vi "Group Modules.vi"(8 "error in":errorcluster, 10 "Item Names":string[](array[string]), 11 "json class out":refnum<class "Build_Javier_Lopez_lib_Configuration_Filejson class.lvclass">) -> (0 "error out":errorcluster, 2 "Enum":T1(c390))   [LabVIEW 2021]
uses:
  <vilib>/Javier Lopez/Configuration File/Json Element/Build_Javier_Lopez_lib_Configuration_Filejson class.lvclass
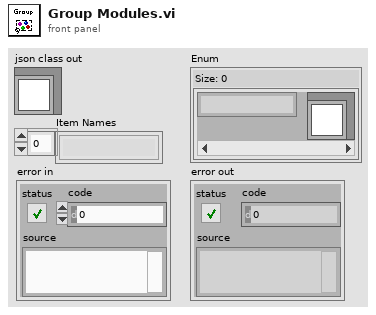
[diagram p1: front panel]
types:
  T1 = map{string, refnum<class "Build_Javier_Lopez_lib_Configuration_Filejson class.lvclass">}
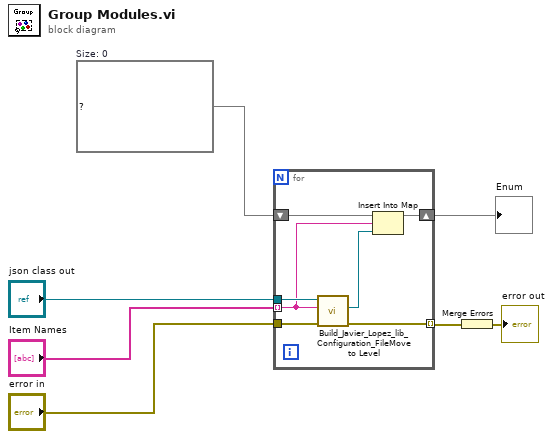
[diagram p0: block diagram]
diagram:
  w6 = T1 {}  # Size: 0
  n1 = for {
    shift-right: [w14] -> w7
    shift-left: w6 -> [w13]
    tunnel: "json class out" -> [w12]
    tunnel: "error in" -> [w11]
    tunnel: "Item Names" -> [w9] mode=indexing
    tunnel: [w8] -> w2 mode=indexing
    n2 = call-dynamic "Build_Javier_Lopez_lib_Configuration_FileMove to Level.vi"("error in (no error)"=w11, "Element"=w9, "json class in"=w12) -> ("error out"=w8:errorcluster, "New json class"=w10:refnum<class "Build_Javier_Lopez_lib_Configuration_Filejson class.lvclass">)  [unwired: 6 in, 1 out]
    n3 = Insert Into Map(map in=w13, key=w9, value=w10) -> (map out=w14:T1)  [unwired: 2 out]
  }
  "Enum" <- w7
  n4 = Merge Errors(w2) -> (→"error out":errorcluster)
